vi "waveform_length.vi"(1 "WL":dbl, 2 "Cola WL":refnum<queue>, 3 "Datos entrada":refnum<queue>) -> (0 "WL 2":dbl)   [LabVIEW 2016]
doc: "Computa el waveform length a partir de una cola de vectores que contiene los datos de entrada y de una cola de numeros que contiene los valores que se suman al acumulado del wafeform length y que además indica el tamaño de la ventana que se utiliza para llevar a cabo este calculo."
panel:
  in  "Last Data":dbl
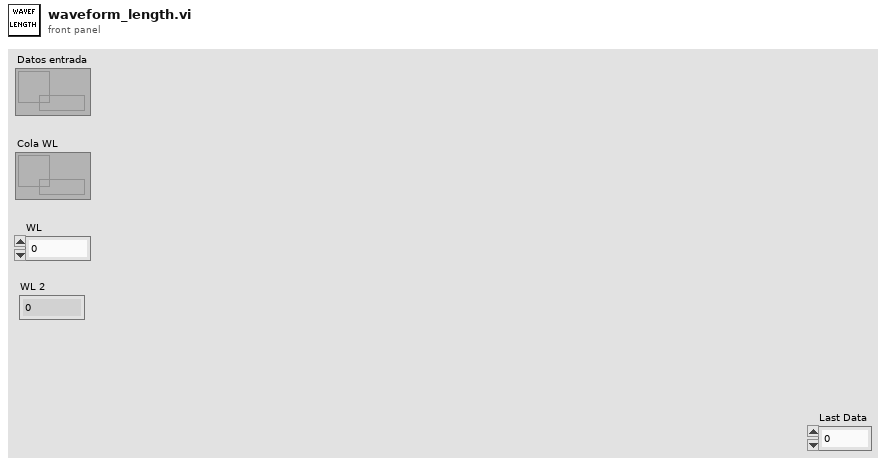
[diagram p1: front panel]
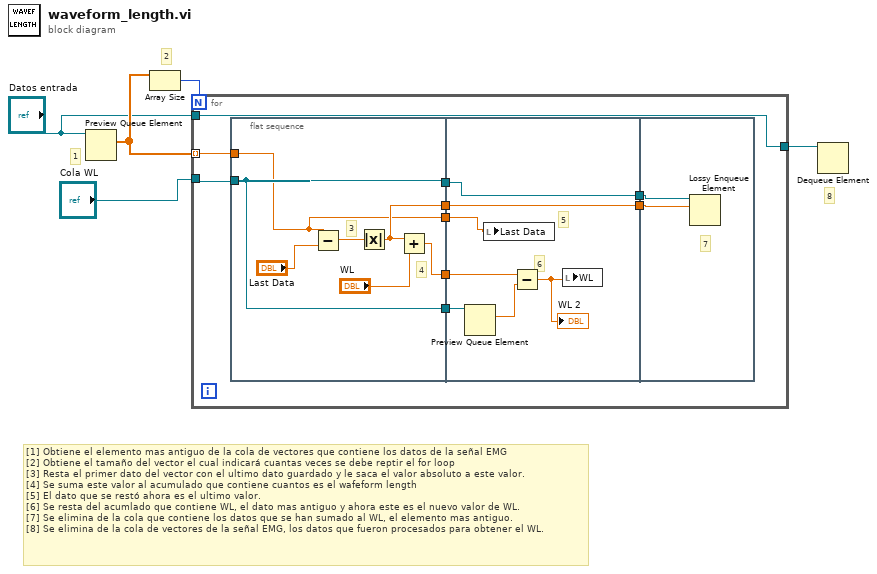
[diagram p0: block diagram]
diagram:
  # "8"
  # "2"
  # "1"
  # "[1] Obtiene el elemento mas antiguo de la cola de vectores que contiene los datos de la señal EMG\n[2] Obtiene el tamaño del vector el cual indicará cuantas veces se debe reptir el for loop\n[3] Resta el primer dato del vector con el ultimo dato guardado y le saca el valor absoluto a este valor.\n[4] Se suma este valor al acumulado que contiene cuantos es el wafeform length\n[5] El dato que se restó ahora es el ultimo valor.\n[6] Se resta del acumlado que contiene WL, el dato mas antiguo y ahora este es el nuevo valor de WL.\n[7] Se elimina de la cola que contiene los datos que se han sumado al WL, el elemento mas antiguo.\n[8] Se elimina de la cola de vectores de la señal EMG, los datos que fueron procesados para obtener el WL."
  n1 = Preview Queue Element(queue="Datos entrada") -> (element=w3:dbl[])  [unwired: 2 in, 3 out]
  n2 = Array Size(array=w3) -> (size(s)=w5:i32)
  n3 = for {
    N: w5 -> [_]
    tunnel: "Cola WL" -> [w15]
    tunnel: w3 -> [w7] mode=indexing
    tunnel: "Datos entrada" -> [w6]
    tunnel: [w6] -> w1
    n4 = flat-sequence {
      tunnel: [w16] -> w14
      tunnel: [w19] -> w13
      tunnel: w15 -> [w18]
      tunnel: [w18] -> w12
      tunnel: [w18] -> w11
      tunnel: [w17] -> w10
      tunnel: w7 -> [w16]
      tunnel: w14 -> [w29]
      tunnel: w13 -> [w28]
      tunnel: w12 -> [w26]
      tunnel: w11 -> [w25]
      tunnel: [w25] -> w9
      tunnel: w10 -> [w24]
      tunnel: [w24] -> w8
      tunnel: w9 -> [w31]
      tunnel: w8 -> [w30]
      frame #0 {
        # "4"
        # "3"
        n5 = Subtract(x=w16, y="Last Data") -> (x-y=w22:dbl)
        n6 = Absolute Value(x=w22) -> (abs(x)=w17:dbl)
        n7 = Add(x=w17, y="WL") -> (x+y=w19:dbl)
      }
      frame #1 {
        # "6"
        # "5"
        n8 = Preview Queue Element(queue=w26) -> (element=w27:dbl)  [unwired: 2 in, 3 out]
        n9 = local write "Last Data"(w29) -> ()
        n10 = Subtract(x=w28, y=w27) -> (x-y=w23:dbl)
        "WL 2" <- w23
        n11 = local write "WL"(w23) -> ()
      }
      frame #2 {
        # "7"
        n12 = Lossy Enqueue Element(queue=w31, element=w30) -> ()  [unwired: 1 in, 4 out]
      }
    }
  }
  n13 = Dequeue Element(queue=w1) -> ()  [unwired: 2 in, 4 out]
